vi "R45_1-FPGA.vi"() -> ()   [LabVIEW 2016]
uses:
  control vi/controls/Faraday Cup Readback.ctl
  control vi/controls/Aperture Readback.ctl
  control vi/controls/Glassman Readback.ctl
  control vi/controls/Glassman Control.ctl
  <vilib>/LabVIEW Targets/FPGA/cRIO/shared/nicrio_ModuleControls/nicrio_cRIO-9871_BaudRateEnum.ctl
  <vilib>/LabVIEW Targets/FPGA/cRIO/shared/nicrio_ModuleControls/nicrio_cRIO-9871_ParityEnum.ctl
  <vilib>/LabVIEW Targets/FPGA/cRIO/shared/nicrio_ModuleControls/nicrio_cRIO-9871_StopBitsEnum.ctl
  <vilib>/LabVIEW Targets/FPGA/cRIO/shared/nicrio_ModuleControls/nicrio_cRIO-9871_DataBitsEnum.ctl
  <vilib>/Platform/TimedLoop/XDataNode/timing_clust.ctl
  <vilib>/Platform/TimedLoop/XDataNode/nitl_modes.ctl
  <vilib>/Platform/TimedLoop/XDataNode/wakeup.ctl
  <vilib>/rvi/FXPMathLib/basic elements/FxpIntAccumulator/subVIs/nifxpmath_IntAccumulator_SimConfig.ctl
  <vilib>/rvi/Emulation/niFpgaGetClockAttributes.vi
  <vilib>/rvi/Emulation/niFpgaSctlEmulationGetInTimedLoop.vi
  <vilib>/rvi/Emulation/niFpgaEmulationReportErrorSimple.vi
  <vilib>/rvi/eio/common/nirviEmuTemplateMethod_errors.vi
  <vilib>/rvi/Emulation/niFpgaCriticalErrorInLSC.vi
  <vilib>/rvi/Analysis/common/codeGenErrors/XNode/niFpgaXNodeCodeGenErrorHandle.vi
  <vilib>/rvi/FXPMathLib/basic elements/FxpIntAccumulator/simVIs/DllFxpIntAccumulator_sub.vi
  <vilib>/rvi/eio/common/nirviEmuTemplatePropertySet_errors.vi
  <vilib>/eio/EIONode/EIONode.xnode
  <vilib>/rvi/Analysis/measure/dc-rms/XNode/niFpgaDC-RMS.xnode
  <vilib>/Platform/TimedLoop/XDataNode/XDataNode.xnode
  <vilib>/rvi/FXPMathLib/basic elements/FxpIntAccumulator/XNode/nifxpmath_IntAccumulator.xnode
  <vilib>/rvi/FXPMathLib/FxpMul/XNode/nifxpmath_Multiplier.xnode
  <vilib>/eio/EIOPropertyNode/EIOPropertyNode.xnode
  <vilib>/eio/EIOMethodNode/EIOMethodNode.xnode
  <vilib>/Platform/TimedLoop/XDataNode/XDNodeRunTimeDep.lvlib
  <vilib>/rvi/FXPMathLib/sim/FxpSim.dll
  <vilib>/rvi/eio/common/nirviEmuTemplatePropertyGet_errors.vi
  <vilib>/rvi/eio/common/nirviEmuTemplatePropertyGet_noerrors.vi
  <vilib>/rvi/eio/common/nirviEmuTemplatePropertySet_noerrors.vi
panel:
  out "2nd stage temp":u8[](array[numeric])
  out "Time since repurge":u8[](array[numeric])
  out "Cryo pump error":errorcluster
  out "Cryo 1st stage temp":u8[](array[numeric])
  out "Cryo On-time":u8[](array[numeric])
  out "Cryo status":u8[](array[numeric])
  in  "RT error":bool
  in  "Switch Mag Aperture actuator":bool
  in  "Switch Mag FC actuator":bool
  out "Cup-Aperture Control Loop Error":errorcluster
  out "Vac Cluster 1 Ion Gauge 2":u8[](array[numeric])
  out "Vac Cluster 1 Convectron 2":u8[](array[numeric])
  out "Vac Cluster 1 Convectron 1":u8[](array[numeric])
  out "Vac Cluster 1 Ion Gauge 1":u8[](array[numeric])
  out "Vacuum Gauge 1 error":errorcluster
  in  "Right Steerer Voltage set":T1
  in  "Down Steerer Voltage set":T1
  out "HV Control error":errorcluster
  in  "Up Steerer Voltage set":T1
  in  "Left Steerer Voltage set":T1
  out "Right Steerer readback":T2
  out "Left Steerer readback":T2
  out "Down Steerer readback":T2
  out "Up Steerer readback":T2
  out "HV readback error":errorcluster
  out "Position-Sensor readback error":errorcluster
  out "Switch Mag Aperture Position":T3
  out "Switch Mag FC Position":T4
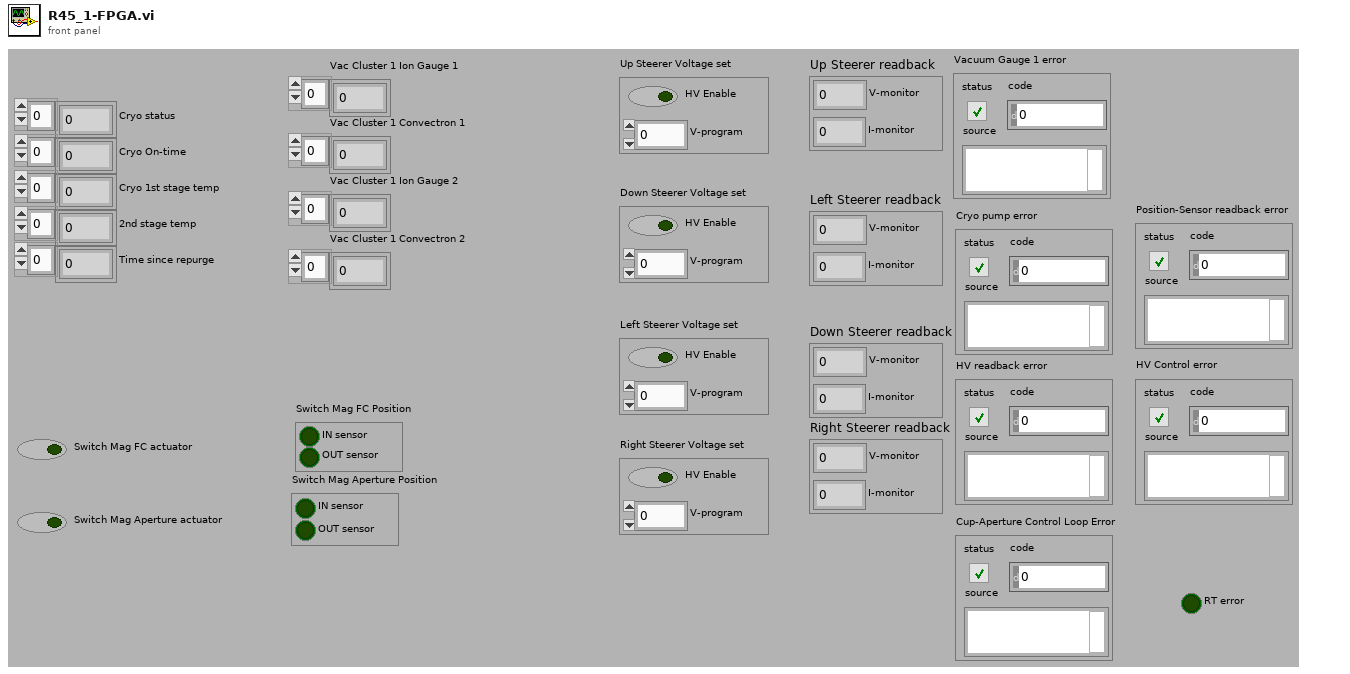
[diagram p1: front panel]
types:
  T1 = typedef "Glassman Control.ctl" = cluster{"V-program":fxp<+/-,16,5>, "HV Enable":bool}
  T2 = typedef "Glassman Readback.ctl" = cluster{"I-monitor":fxp<+/-,16,5>, "V-monitor":fxp<+/-,16,5>}
  T3 = typedef "Aperture Readback.ctl" = cluster{"IN sensor":bool, "OUT sensor":bool}
  T4 = typedef "Faraday Cup Readback.ctl" = cluster{"IN sensor":bool, "OUT sensor":bool}
  T5 = typedef "nicrio_cRIO-9871_ParityEnum.ctl" = enum8{"None", "Odd", "Even", "Mark", "Space"}
  T6 = typedef "nicrio_cRIO-9871_StopBitsEnum.ctl" = enum8{"1", "1.5", "2"}
  T7 = typedef "nicrio_cRIO-9871_DataBitsEnum.ctl" = enum8{"5", "6", "7", "8"}
  T8 = typedef "nicrio_cRIO-9871_BaudRateEnum.ctl" = enum16{"75 bps", "110 bps", "134 bps", "150 bps", "300 bps", "600 bps", "1200 bps", "1800 bps", "2400 bps", "4800 bps", "7200 bps", "9600 bps", "14.4 kbps", "19.2 kbps", "28.8 kbps", "38.4 kbps", "57.6 kbps", "115.2 kbps", "230.4 kbps", "460.8 kbps", "921.6 kbps"}
  T9 = typedef "XDNodeRunTimeDep.lvlib/timing_clust.ctl" = cluster{"Expected End [f-1]":u64, "Actual End [f-1]":u64, "Finished Late? [f-1]":bool, "Expected End [i-1]":u64, "Actual End [i-1]":u64, "Finished Late? [i-1]":bool, "Expected Start [i]":u64, "Actual Start [i]":u64, "Expected Start [f]":u64, "Actual Start [f]":u64, "Source Name":string, "Structure Name":string, "Period":i64, "Deadline":i64, "Offset":i64, "Start":i64, "Priority":i32, "Timeout":i32, "Mode":T10, "Wakeup Reason":T11, "Error":errorcluster, "Source Type":string, "Secondary Source Type":string, "Global End Time":u64, "Global Start Time":u64, "Frame Duration":u64, "Iteration Duration":u64, "Assigned CPU":i32, "I/O Scan Engine Mode":u32}
  T10 = typedef "XDNodeRunTimeDep.lvlib/nitl_modes.ctl" = enum32{"No Change", "Process missed periods, maintain original phase", "Discard missed periods, maintain original phase", "Process missed periods, ignore original phase", "Discard missed periods, ignore original phase"}
  T11 = typedef "XDNodeRunTimeDep.lvlib/wakeup.ctl" = enum32{"Normal", "Aborted", "Asynchronous wakeup", "Timing source error", "Timed loop error", "Timeout"}
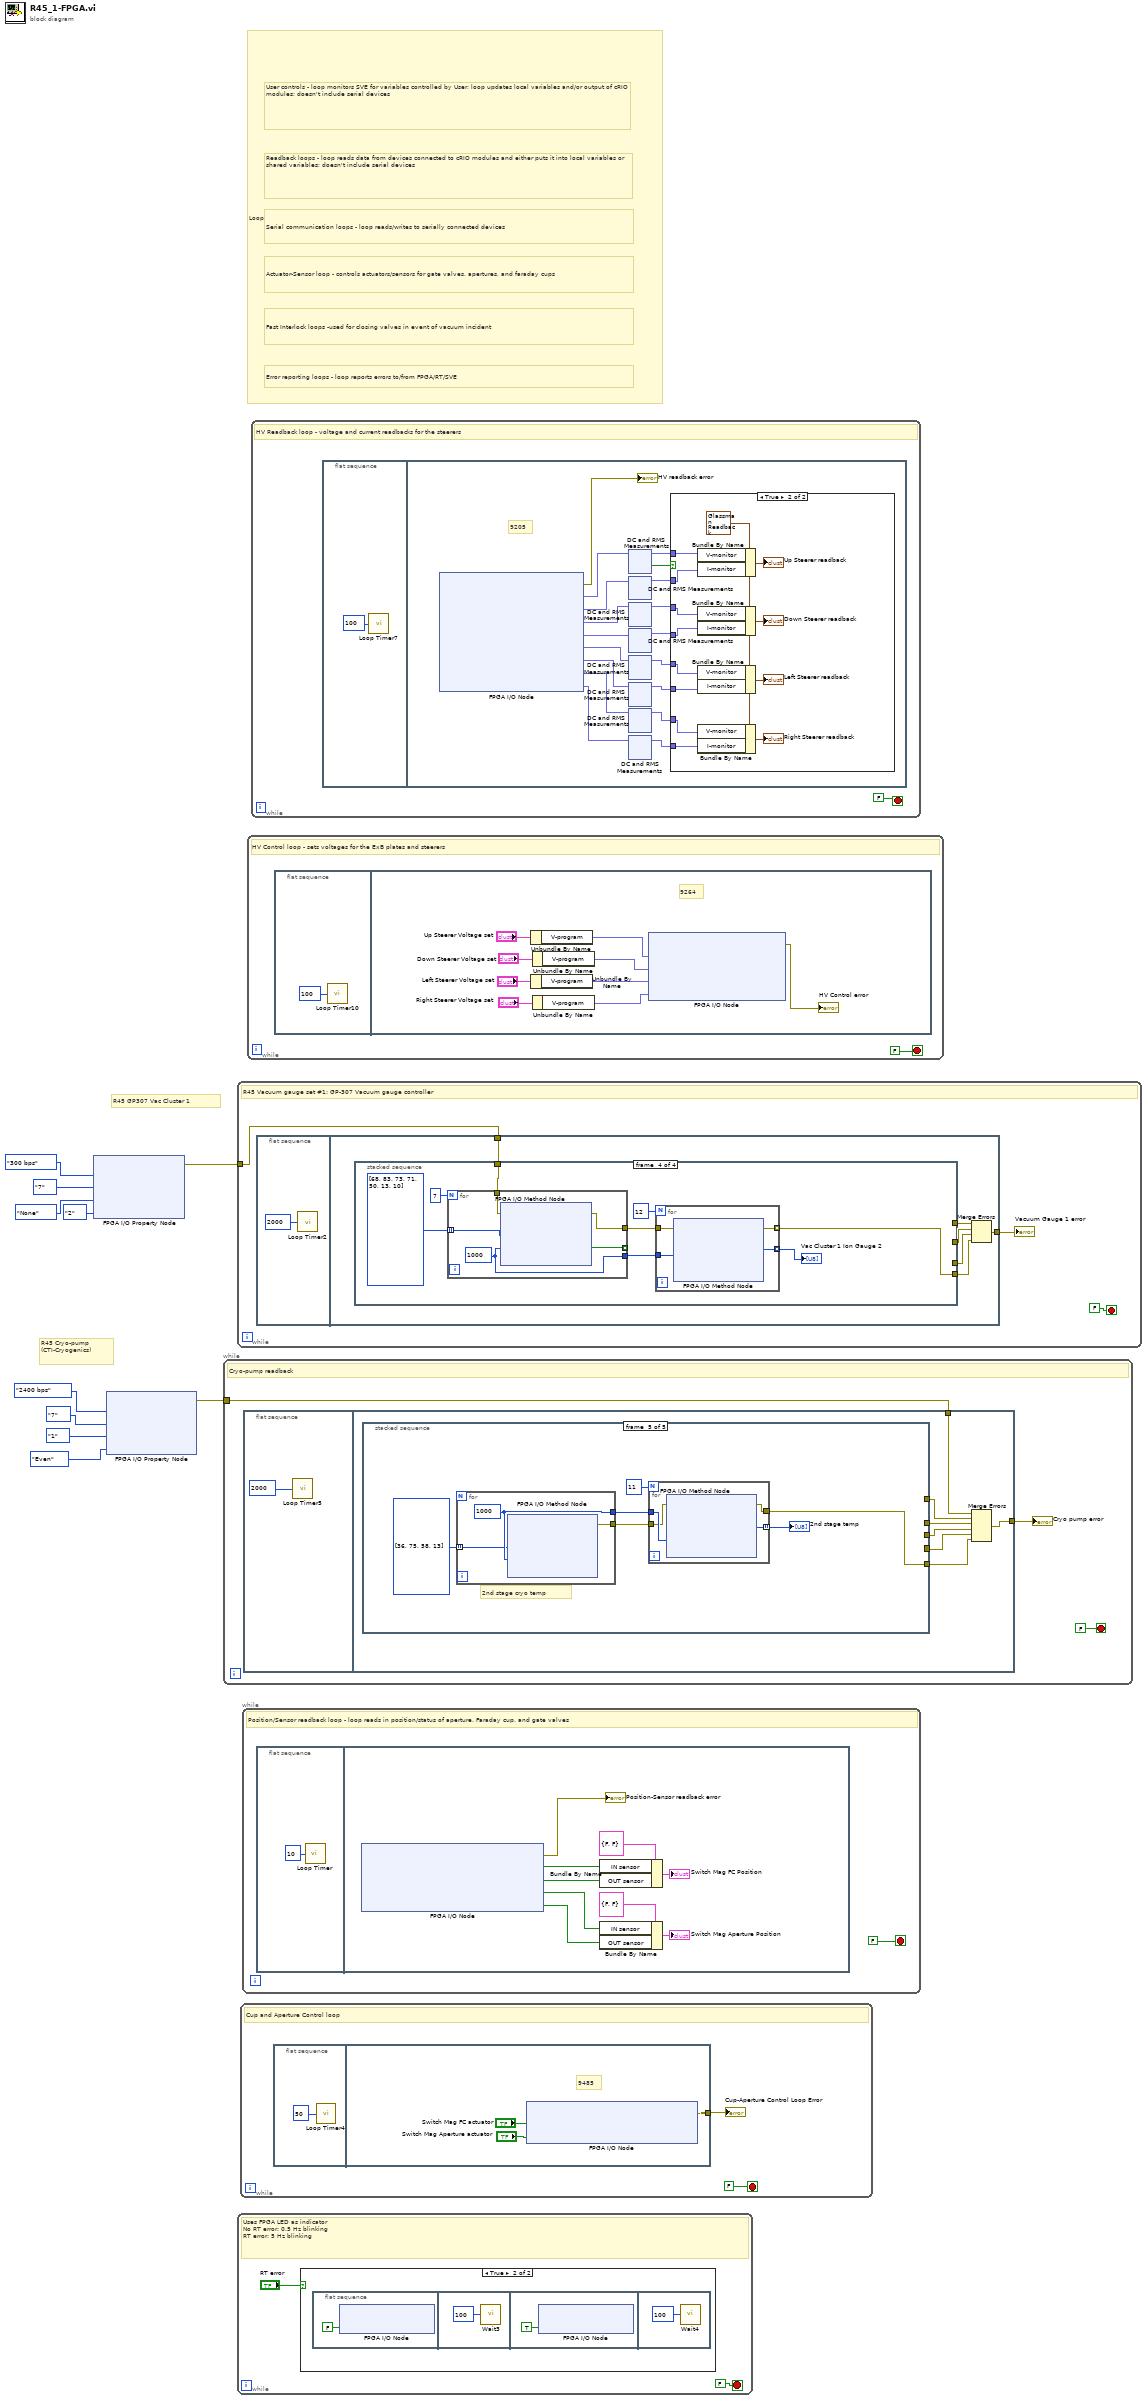
[diagram p0: block diagram]
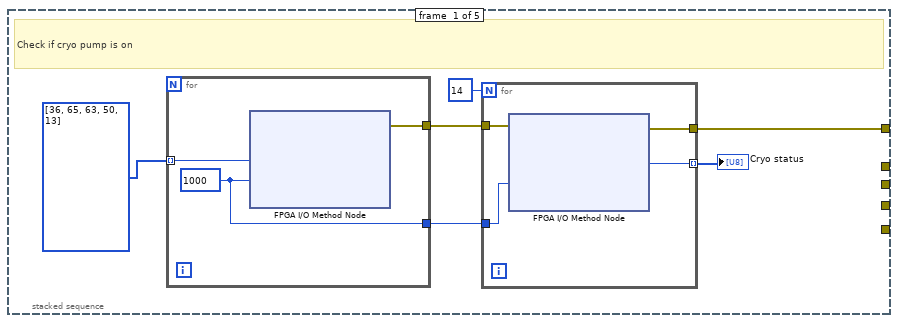
[diagram p2: hidden frame]
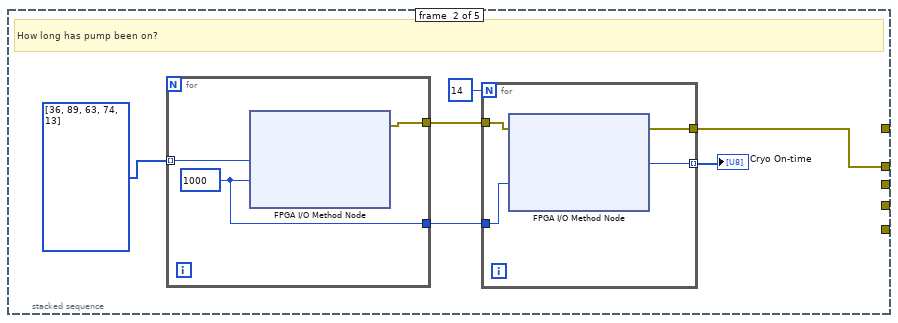
[diagram p3: hidden frame]
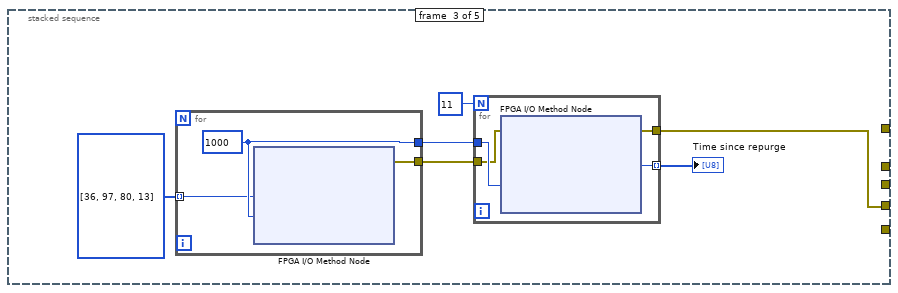
[diagram p4: hidden frame]
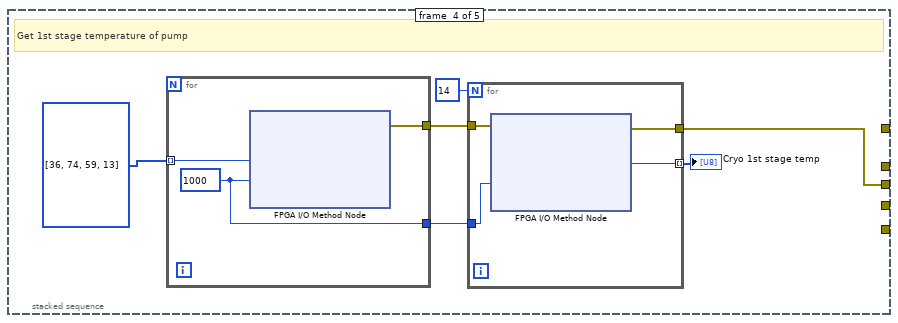
[diagram p5: hidden frame]
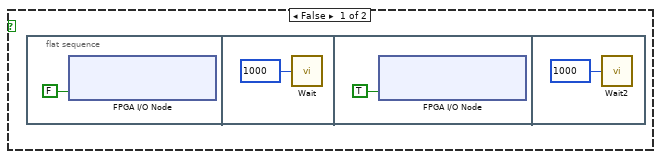
[diagram p6: hidden frame]
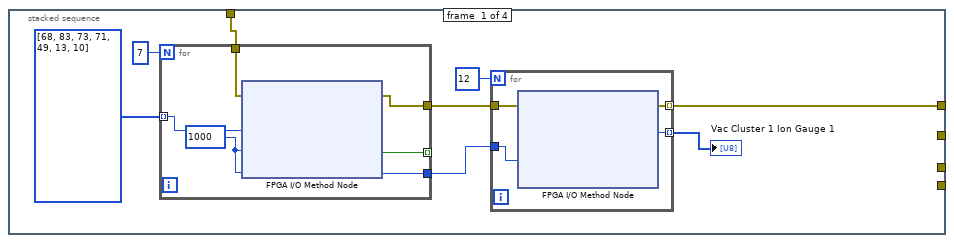
[diagram p7: hidden frame]
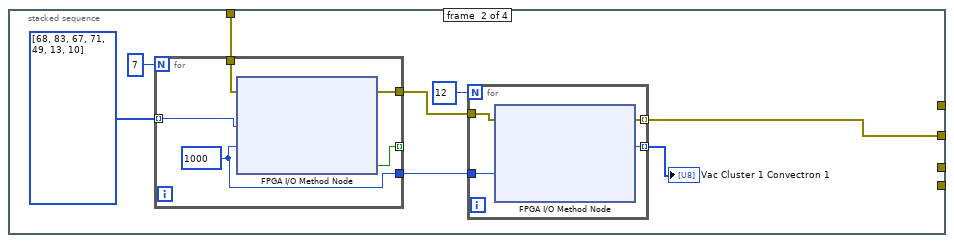
[diagram p8: hidden frame]
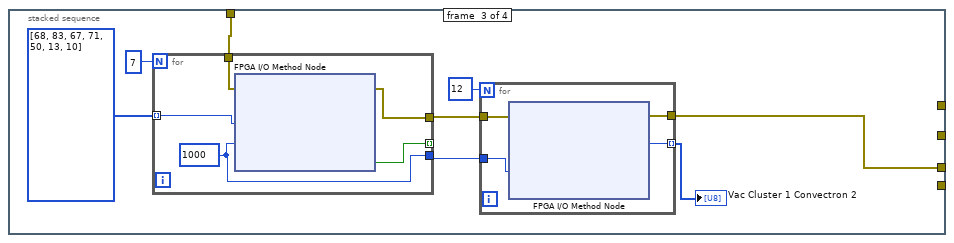
[diagram p9: hidden frame]
diagram:
  # "Actuator-Sensor loop - controls actuators/sensors for gate valves, apertures, and faraday cups"
  # "R45 Cryo-pump\n(CTI-Cryogenics)"
  # "R45 GP307 Vac Cluster 1"
  # "Fast Interlock loops -used for closing valves in event of vacuum incident"
  # "Error reporting loops - loop reports errors to/from FPGA/RT/SVE"
  # "Serial communication loops - loop reads/writes to serially connected devices"
  # "Readback loops - loop reads data from devices connected to cRIO modules and either puts it into local variables or shared variables; doesn't include serial devices"
  # "User controls - loop monitors SVE for variables controlled by User; loop updates local variables and/or output of cRIO modules; doesn't include serial devices"
  # "Loop legend - loops are color coded by responsibility"
  n1 = xnode "FPGA I/O Property Node"("Baud Rate"=nicrio_cRIO-9871_BaudRateEnum."300 bps", "Data Bits"=nicrio_cRIO-9871_DataBitsEnum."7", "Parity"=nicrio_cRIO-9871_ParityEnum."None", "Stop Bits"=nicrio_cRIO-9871_StopBitsEnum."2") -> ("error out"=w6:errorcluster)  [unwired: 2 in, 1 out]
  n2 = xnode "FPGA I/O Property Node"("Baud Rate"=nicrio_cRIO-9871_BaudRateEnum."2400 bps", "Data Bits"=nicrio_cRIO-9871_DataBitsEnum."7", "Stop Bits"=nicrio_cRIO-9871_StopBitsEnum."1", "Parity"=nicrio_cRIO-9871_ParityEnum."Even") -> ("error out"=w1:errorcluster)  [unwired: 2 in, 1 out]
  n3 = while {
    tunnel: w1 -> [w12]
    stop <- FALSE stop-if-true
    # "Cryo-pump readback"
    n4 = flat-sequence {
      tunnel: w12 -> [w21]
      tunnel: [w20] -> w11
      frame #0 {
        n5 = call "Loop Timer5"("Count(mSec)"=u32 2000) -> ()  [unwired: 1 out]
      }
      frame #1 {
        n6 = stacked-sequence {
          tunnel: [_ w35 _ _ _] -> w19
          tunnel: [w22 _ _ _ _] -> w18
          tunnel: [_ _ _ w61 _] -> w17
          tunnel: [_ _ w48 _ _] -> w16
          tunnel: [_ _ _ _ w74] -> w15
          frame #0 {
            # "Check if cryo pump is on"
            n7 = for {
              tunnel: u8[] [36, 65, 63, 50, 13] ("unsigned byte array") -> [w34] mode=indexing
              tunnel: [w33] -> w25
              tunnel: [w32] -> w23
              w33 = 1000 ("Timeout (ms)")
              n8 = xnode "FPGA I/O Method Node"("Data"=w34, "Timeout (ms)"=w33) -> ("error out"=w32:errorcluster)  [unwired: 2 in, 2 out]
            }
            n9 = for {
              N: 14 -> [_]
              tunnel: [w31] -> w27 mode=indexing
              tunnel: w25 -> [w30]
              tunnel: w23 -> [w29]
              tunnel: [w28] -> w22
              n10 = xnode "FPGA I/O Method Node"("error in"=w29, "Timeout (ms)"=w30) -> ("error out"=w28:errorcluster, "Data"=w31:u8)  [unwired: 1 in, 2 out]
            }
            "Cryo status" <- w27
          }
          frame #1 {
            # "How long has pump been on?"
            n11 = for {
              tunnel: u8[] [36, 89, 63, 74, 13] ("unsigned byte array") -> [w47] mode=indexing
              tunnel: [w46] -> w38
              tunnel: [w45] -> w36
              w46 = 1000 ("Timeout (ms)")
              n12 = xnode "FPGA I/O Method Node"("Data"=w47, "Timeout (ms)"=w46) -> ("error out"=w45:errorcluster)  [unwired: 2 in, 2 out]
            }
            n13 = for {
              N: 14 -> [_]
              tunnel: [w44] -> w40 mode=indexing
              tunnel: w38 -> [w43]
              tunnel: w36 -> [w42]
              tunnel: [w41] -> w35
              n14 = xnode "FPGA I/O Method Node"("error in"=w42, "Timeout (ms)"=w43) -> ("error out"=w41:errorcluster, "Data"=w44:u8)  [unwired: 1 in, 2 out]
            }
            "Cryo On-time" <- w40
          }
          frame #2 {
            n15 = for {
              tunnel: [w60] -> w53
              tunnel: u8[] [36, 97, 80, 13] ("unsigned byte array") -> [w58] mode=indexing
              tunnel: [w59] -> w49
              w60 = 1000 ("Timeout (ms)")
              n16 = xnode "FPGA I/O Method Node"("Data"=w58, "Timeout (ms)"=w60) -> ("error out"=w59:errorcluster)  [unwired: 2 in, 2 out]
            }
            n17 = for {
              N: 11 -> [_]
              tunnel: w53 -> [w57]
              tunnel: [w56] -> w50 mode=indexing
              tunnel: w49 -> [w55]
              tunnel: [w54] -> w48
              n18 = xnode "FPGA I/O Method Node"("error in"=w55, "Timeout (ms)"=w57) -> ("error out"=w54:errorcluster, "Data"=w56:u8)  [unwired: 1 in, 2 out]
            }
            "Time since repurge" <- w50
          }
          frame #3 {
            # "Get 1st stage temperature of pump"
            n19 = for {
              tunnel: u8[] [36, 74, 59, 13] ("unsigned byte array") -> [w73] mode=indexing
              tunnel: [w72] -> w64
              tunnel: [w71] -> w62
              w72 = 1000 ("Timeout (ms)")
              n20 = xnode "FPGA I/O Method Node"("Data"=w73, "Timeout (ms)"=w72) -> ("error out"=w71:errorcluster)  [unwired: 2 in, 2 out]
            }
            n21 = for {
              N: 14 -> [_]
              tunnel: [w70] -> w66 mode=indexing
              tunnel: w64 -> [w69]
              tunnel: w62 -> [w68]
              tunnel: [w67] -> w61
              n22 = xnode "FPGA I/O Method Node"("error in"=w68, "Timeout (ms)"=w69) -> ("error out"=w67:errorcluster, "Data"=w70:u8)  [unwired: 1 in, 2 out]
            }
            "Cryo 1st stage temp" <- w66
          }
          frame #4 {
            # "2nd stage cryo temp"
            n23 = for {
              tunnel: [w86] -> w79
              tunnel: u8[] [36, 75, 58, 13] ("unsigned byte array") -> [w85] mode=indexing
              tunnel: [w84] -> w75
              w86 = 1000 ("Timeout (ms)")
              n24 = xnode "FPGA I/O Method Node"("Data"=w85, "Timeout (ms)"=w86) -> ("error out"=w84:errorcluster)  [unwired: 2 in, 2 out]
            }
            n25 = for {
              N: 11 -> [_]
              tunnel: w79 -> [w83]
              tunnel: [w82] -> w76 mode=indexing
              tunnel: w75 -> [w81]
              tunnel: [w80] -> w74
              n26 = xnode "FPGA I/O Method Node"("error in"=w81, "Timeout (ms)"=w83) -> ("error out"=w80:errorcluster, "Data"=w82:u8)  [unwired: 1 in, 2 out]
            }
            "2nd stage temp" <- w76
          }
        }
        n27 = Merge Errors(w21, w18, w19, w17, w16, w15) -> (w20:errorcluster)
      }
    }
    "Cryo pump error" <- w11
  }
  n28 = while {
    tunnel: w6 -> [w88]
    stop <- FALSE stop-if-true
    # "R45 Vacuum gauge set #1: GP-307 Vacuum gauge controller"
    n29 = flat-sequence {
      tunnel: w88 -> [w96]
      tunnel: [w91] -> w87
      frame #0 {
        n30 = call "Loop Timer2"("Count(mSec)"=u32 2000 ("Count(Ticks)")) -> ()  [unwired: 1 out]
      }
      frame #1 {
        n31 = stacked-sequence {
          tunnel: [_ _ w133 _] -> w93
          tunnel: [_ _ _ w149] -> w92
          tunnel: w96 -> [w99 w116 w131 w148]
          tunnel: [w97 _ _ _] -> w95
          tunnel: [_ w115 _ _] -> w94
          frame #0 {
            n32 = for {
              N: 7 -> [_]
              tunnel: [w113] -> w100
              tunnel: [w112] -> _ mode=indexing
              tunnel: u8[] [68, 83, 73, 71, 49, 13, 10] ("unsigned byte array") -> [w111] mode=indexing
              tunnel: w99 -> [w110]
              tunnel: [w109] -> w98
              w113 = 1000 ("Timeout (ms)")
              n33 = xnode "FPGA I/O Method Node"("error in"=w110, "Data"=w111, "Timeout (ms)"=w113) -> ("error out"=w109:errorcluster, "Timed Out"=w112:bool)  [unwired: 1 in, 1 out]
            }
            n34 = for {
              N: 12 -> [_]
              tunnel: w100 -> [w108]
              tunnel: [w107] -> w101 mode=indexing
              tunnel: w98 -> [w106]
              tunnel: [w105] -> w97 mode=indexing
              n35 = xnode "FPGA I/O Method Node"("error in"=w106, "Timeout (ms)"=w108) -> ("error out"=w105:errorcluster, "Data"=w107:u8)  [unwired: 1 in, 2 out]
            }
            "Vac Cluster 1 Ion Gauge 1" <- w101
          }
          frame #1 {
            n36 = for {
              N: 7 -> [_]
              tunnel: [w129] -> w121
              tunnel: [w128] -> _ mode=indexing
              tunnel: u8[] [68, 83, 67, 71, 49, 13, 10] ("unsigned byte array") -> [w130] mode=indexing
              tunnel: w116 -> [w127]
              tunnel: [w126] -> w114
              w129 = 1000 ("Timeout (ms)")
              n37 = xnode "FPGA I/O Method Node"("error in"=w127, "Data"=w130, "Timeout (ms)"=w129) -> ("error out"=w126:errorcluster, "Timed Out"=w128:bool)  [unwired: 1 in, 1 out]
            }
            n38 = for {
              N: 12 -> [_]
              tunnel: w121 -> [w125]
              tunnel: [w124] -> w117 mode=indexing
              tunnel: w114 -> [w123]
              tunnel: [w122] -> w115 mode=indexing
              n39 = xnode "FPGA I/O Method Node"("error in"=w123, "Timeout (ms)"=w125) -> ("error out"=w122:errorcluster, "Data"=w124:u8)  [unwired: 1 in, 2 out]
            }
            "Vac Cluster 1 Convectron 1" <- w117
          }
          frame #2 {
            n40 = for {
              N: 7 -> [_]
              tunnel: [w145] -> w138
              tunnel: [w146] -> _ mode=indexing
              tunnel: u8[] [68, 83, 67, 71, 50, 13, 10] ("unsigned byte array") -> [w147] mode=indexing
              tunnel: [w144] -> w134
              tunnel: w131 -> [w143]
              w145 = 1000 ("Timeout (ms)")
              n41 = xnode "FPGA I/O Method Node"("error in"=w143, "Data"=w147, "Timeout (ms)"=w145) -> ("error out"=w144:errorcluster, "Timed Out"=w146:bool)  [unwired: 1 in, 1 out]
            }
            n42 = for {
              N: 12 -> [_]
              tunnel: w138 -> [w142]
              tunnel: [w141] -> w132 mode=indexing
              tunnel: w134 -> [w140]
              tunnel: [w139] -> w133
              n43 = xnode "FPGA I/O Method Node"("error in"=w140, "Timeout (ms)"=w142) -> ("error out"=w139:errorcluster, "Data"=w141:u8)  [unwired: 1 in, 2 out]
            }
            "Vac Cluster 1 Convectron 2" <- w132
          }
          frame #3 {
            n44 = for {
              N: 7 -> [_]
              tunnel: [w162] -> w155
              tunnel: [w164] -> _ mode=indexing
              tunnel: u8[] [68, 83, 73, 71, 50, 13, 10] ("unsigned byte array") -> [w163] mode=indexing
              tunnel: [w161] -> w150
              tunnel: w148 -> [w160]
              w162 = 1000 ("Timeout (ms)")
              n45 = xnode "FPGA I/O Method Node"("error in"=w160, "Data"=w163, "Timeout (ms)"=w162) -> ("error out"=w161:errorcluster, "Timed Out"=w164:bool)  [unwired: 1 in, 1 out]
            }
            n46 = for {
              N: 12 -> [_]
              tunnel: w155 -> [w159]
              tunnel: [w158] -> w151 mode=indexing
              tunnel: w150 -> [w157]
              tunnel: [w156] -> w149 mode=indexing
              n47 = xnode "FPGA I/O Method Node"("error in"=w157, "Timeout (ms)"=w159) -> ("error out"=w156:errorcluster, "Data"=w158:u8)  [unwired: 1 in, 2 out]
            }
            "Vac Cluster 1 Ion Gauge 2" <- w151
          }
        }
        n48 = Merge Errors(w95, w94, w93, w92) -> (w91:errorcluster)
      }
    }
    "Vacuum Gauge 1 error" <- w87
  }
  n49 = while {
    stop <- FALSE stop-if-true
    # "Uses FPGA LED as indicator\nNo RT error: 0.5 Hz blinking\nRT error: 5 Hz blinking"
    n50 = case shown="True" "RT error" {
      frame False {
        n51 = flat-sequence {
          frame #0 {
            n52 = xnode "FPGA I/O Node"("USER FPGA LED"=FALSE ("FPGA LED")) -> ()  [unwired: 1 in, 1 out]
          }
          frame #1 {
            n53 = call "Wait"("Count(mSec)"=u16 1000) -> ()  [unwired: 1 out]
          }
          frame #2 {
            n54 = xnode "FPGA I/O Node"("USER FPGA LED"=TRUE ("FPGA LED")) -> ()  [unwired: 1 in, 1 out]
          }
          frame #3 {
            n55 = call "Wait2"("Count(mSec)"=u16 1000) -> ()  [unwired: 1 out]
          }
        }
      }
      frame True {
        n56 = flat-sequence {
          frame #0 {
            n57 = xnode "FPGA I/O Node"("USER FPGA LED"=FALSE ("FPGA LED")) -> ()  [unwired: 1 in, 1 out]
          }
          frame #1 {
            n58 = call "Wait3"("Count(mSec)"=u16 100) -> ()  [unwired: 1 out]
          }
          frame #2 {
            n59 = xnode "FPGA I/O Node"("USER FPGA LED"=TRUE ("FPGA LED")) -> ()  [unwired: 1 in, 1 out]
          }
          frame #3 {
            n60 = call "Wait4"("Count(mSec)"=u16 100) -> ()  [unwired: 1 out]
          }
        }
      }
    }
  }
  n61 = while {
    stop <- FALSE stop-if-true
    # "Cup and Aperture Control loop"
    n62 = flat-sequence {
      tunnel: [w178] -> w175
      frame #0 {
        n63 = call "Loop Timer4"("Count(mSec)"=u32 50 ("Count(Ticks)")) -> ()  [unwired: 1 out]
      }
      frame #1 {
        # "9485"
        n64 = xnode "FPGA I/O Node"("Switch Magnet FC Actuator"="Switch Mag FC actuator", "Switch Magnet Aperture Actuator"="Switch Mag Aperture actuator") -> ("error out"=w178:errorcluster)  [unwired: 3 in, 2 out]
      }
    }
    "Cup-Aperture Control Loop Error" <- w175
  }
  n65 = while {
    stop <- FALSE stop-if-true
    # "Position/Sensor readback loop - loop reads in position/status of aperture, Faraday cup, and gate valves"
    n66 = flat-sequence {
      frame #0 {
        n67 = call "Loop Timer"("Count(uSec)"=u32 10 ("Count(Ticks)")) -> ()  [unwired: 1 out]
      }
      frame #1 {
        n68 = xnode "FPGA I/O Node"() -> ("error out"=→"Position-Sensor readback error":errorcluster, "Switch Magnet FC IN sensor"=w189:bool, "Switch Magnet FC OUT sensor"=w188:bool, "Switch Magnet Aperture IN sensor"=w187:bool, "Switch Magnet Aperture OUT sensor"=w186:bool)  [unwired: 5 in, 4 out]
        n69 = Bundle By Name(cluster=T4 {"IN sensor"=FALSE, "OUT sensor"=FALSE} ("Faraday Cup"), "IN sensor"=w189, "OUT sensor"=w188) -> (→"Switch Mag FC Position":T4)
        n70 = Bundle By Name(cluster=T3 {"IN sensor"=FALSE, "OUT sensor"=FALSE} ("Aperture"), "IN sensor"=w187, "OUT sensor"=w186) -> (→"Switch Mag Aperture Position":T3)
      }
    }
  }
  n71 = while {
    stop <- FALSE stop-if-true
    # "HV Control loop - sets voltages for the ExB plates and steerers"
    n72 = flat-sequence {
      frame #0 {
        n73 = call "Loop Timer10"("Count(mSec)"=u32 100 ("Count(Ticks)")) -> ()  [unwired: 1 out]
      }
      frame #1 {
        # "9264"
        n74 = Unbundle By Name("Up Steerer Voltage set") -> ("V-program"=w200:fxp<+/-,16,5>)
        n75 = Unbundle By Name("Left Steerer Voltage set") -> ("V-program"=w199:fxp<+/-,16,5>)
        n76 = Unbundle By Name("Down Steerer Voltage set") -> ("V-program"=w195:fxp<+/-,16,5>)
        n77 = Unbundle By Name("Right Steerer Voltage set") -> ("V-program"=w194:fxp<+/-,16,5>)
        n78 = xnode "FPGA I/O Node"("Up Steerer Voltage set"=w200, "Down Steerer Voltage set"=w195, "Left Steerer Voltage set"=w199, "Right Steerer Voltage set"=w194) -> ("error out"=→"HV Control error":errorcluster)  [unwired: 5 in, 4 out]
      }
    }
  }
  n79 = while {
    stop <- FALSE stop-if-true
    # "HV Readback loop - voltage and current readbacks for the steerers"
    n80 = flat-sequence {
      frame #0 {
        n81 = call "Loop Timer7"("Count(mSec)"=u32 100 ("Count(Ticks)")) -> ()  [unwired: 1 out]
      }
      frame #1 {
        # "9205"
        n82 = xnode "FPGA I/O Node"() -> ("error out"=→"HV readback error":errorcluster, "Up Steerer Voltage read"=w220:fxp<+/-,26,5>, "Up Steerer Current read"=w218:fxp<+/-,26,5>, "Down Steerer Voltage read"=w217:fxp<+/-,26,5>, "Down Steerer Current read"=w216:fxp<+/-,26,5>, "Left Steerer Voltage read"=w215:fxp<+/-,26,5>, "Left Steerer Current read"=w214:fxp<+/-,26,5>, "Right Steerer Voltage read"=w213:fxp<+/-,26,5>, "Right Steerer Current read"=w212:fxp<+/-,26,5>)  [unwired: 9 in, 8 out]
        n83 = xnode "DC and RMS Measurements"("input data"=w220) -> ("DC"=w222:fxp<+/-,26,5>, "output valid"=w221:bool)  [unwired: 1 in]
        n84 = xnode "DC and RMS Measurements"("input data"=w218) -> ("DC"=w206:fxp<+/-,26,5>)  [unwired: 1 in, 1 out]
        n85 = xnode "DC and RMS Measurements"("input data"=w217) -> ("DC"=w205:fxp<+/-,26,5>)  [unwired: 1 in, 1 out]
        n86 = xnode "DC and RMS Measurements"("input data"=w216) -> ("DC"=w207:fxp<+/-,26,5>)  [unwired: 1 in, 1 out]
        n87 = xnode "DC and RMS Measurements"("input data"=w215) -> ("DC"=w208:fxp<+/-,26,5>)  [unwired: 1 in, 1 out]
        n88 = xnode "DC and RMS Measurements"("input data"=w214) -> ("DC"=w209:fxp<+/-,26,5>)  [unwired: 1 in, 1 out]
        n89 = xnode "DC and RMS Measurements"("input data"=w213) -> ("DC"=w210:fxp<+/-,26,5>)  [unwired: 1 in, 1 out]
        n90 = xnode "DC and RMS Measurements"("input data"=w212) -> ("DC"=w211:fxp<+/-,26,5>)  [unwired: 1 in, 1 out]
        n91 = case shown="True" w221 {
          tunnel: w222 -> [_ w795]
          tunnel: w206 -> [_ w794]
          tunnel: w205 -> [_ w783]
          tunnel: w207 -> [_ w793]
          tunnel: w208 -> [_ w792]
          tunnel: w209 -> [_ w791]
          tunnel: w210 -> [_ w790]
          tunnel: w211 -> [_ w789]
          frame False {
          }
          frame True {
            w784 = T2 {"I-monitor"=0.0, "V-monitor"=0.0} ("Glassman Readback")
            n92 = Bundle By Name(cluster=w784, "V-monitor"=w795, "I-monitor"=w794) -> (→"Up Steerer readback":T2)
            n93 = Bundle By Name(cluster=w784, "V-monitor"=w783, "I-monitor"=w793) -> (→"Down Steerer readback":T2)
            n94 = Bundle By Name(cluster=w784, "V-monitor"=w792, "I-monitor"=w791) -> (→"Left Steerer readback":T2)
            n95 = Bundle By Name(cluster=w784, "V-monitor"=w790, "I-monitor"=w789) -> (→"Right Steerer readback":T2)
          }
        }
      }
    }
  }
